vi "UDP Receiver.vi"() -> ()   [LabVIEW 2015]
doc: "Use this VI with the UDP Sender VI. Run this VI first.\n\nThe UDP protocol differs from TCP in that there is no error-checking with the packets of information that are sent, and thus no guarantee whatsoever that an intended recipient will actually receive a given piece of data.\n\nUDP does offer the ability to \"broadcast\" data across a network--simply specify an IP Address of all ones (255.255.255.255) to attempt to broadcast information network-wide. Keep in mind that routers and other network hardware will generally refuse to forward the broadcast beyond certain points, so the extent of the broadcast will in practice be limited."
panel:
  out "# of Bytes Received":i32
  in  "max bytes/read":i32=548
  in  "Port":u16=61557
  out "Data Received":string
  in  "reset":bool
  in  "stop":bool
  # "Instructions:\n1. Open the UDP Sender.vi\n2. Make sure the Port in this VI and the Remote Port in the UDP Sender.vi are the same.\n3. Adjust the Max Bytes/Read in this VI.\n4. Run this VI first.\n5. Run the UDP Sender second.\n6. Look at the data received and the number of bytes received.\nNote: This VI is built to work with the UDP Sender.vi."
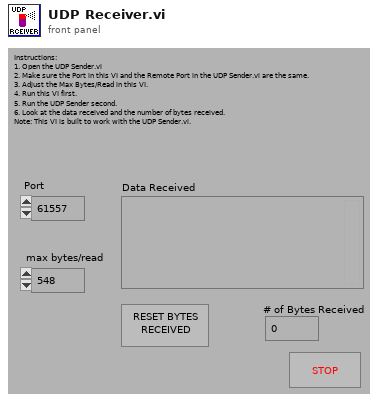
[diagram p1: front panel]
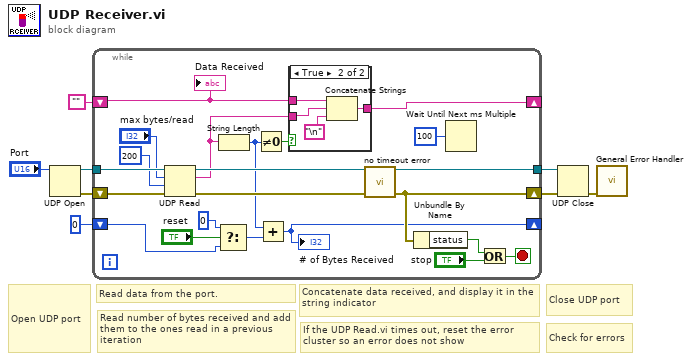
[diagram p0: block diagram]
diagram:
  # "Read number of bytes received and add them to the ones read in a previous iteration"
  # "Check for errors"
  # "Close UDP port"
  # "If the UDP Read.vi times out, reset the error cluster so an error does not show"
  # "Concatenate data received, and display it in the string indicator"
  # "Read data from the port."
  # "Open UDP port"
  n1 = UDP Open(11:"Port") -> (port=w6:refnum<k16>, 0:w7:errorcluster)  [unwired: 4 in, 1 out]
  n2 = while {
    shift-left: "" -> [w12]
    shift-right: [w11] -> _
    shift-left: 0 -> [w17]
    shift-right: [w19] -> _
    tunnel: [w27] -> w5
    tunnel: w6 -> [w28]
    shift-left: w7 -> [w29]
    shift-right: [w21] -> w4
    stop <- w24 stop-if-true
    n3 = UDP Read(connection ID=w28, max size (548)="max bytes/read", timeout ms (25000)=200, 8:w29) -> (data out=w13:string, error out=w22:errorcluster, 3:w27:refnum<k16>)  [unwired: 2 out]
    n4 = Select(t=0, s="reset", f=w17) -> (s? t:f=w16:i32)
    n5 = String Length(string=w13) -> (length=w10:i32)
    n6 = Not Equal To 0?(x=w10) -> (x != 0?=w9:bool)
    n7 = Add(x=w10, y=w16) -> (x+y=w19:i32)
    "# of Bytes Received" <- w19
    n8 = case shown="True" w9 {
      tunnel: w12 -> [w30 w34]
      tunnel: w13 -> [_ w32]
      tunnel: [w30 w33] -> w11
      frame False {
      }
      frame True {
        n9 = Concatenate Strings(w34, w32, "\n" ("Substring")) -> (w33:string)
      }
    }
    n10 = call "no timeout error.vi"("error in (no error)"=w22) -> ("error out"=w21:errorcluster)
    n11 = Unbundle By Name(w21) -> ("status"=w23:bool)
    n12 = Wait Until Next ms Multiple(millisecond multiple=u32 100) -> ()  [unwired: 1 out]
    n13 = Or(x=w23, y="stop") -> (x .or. y?=w24:bool)
    "Data Received" <- w12
  }
  n14 = UDP Close(connection ID=w5, 8:w4) -> (error out=w3:errorcluster)  [unwired: 1 out]
  n15 = call <vilib>:"General Error Handler.vi"("error in (no error)"=w3) -> ()  [unwired: 10 in, 5 out]
